vi "Read Array of Message Info.vi"(8 "error in":errorcluster, 11 "Tx execution unit in":refnum<class "Tx Execution Unit.lvclass">) -> (0 "error out":errorcluster, 2 "array of message info":T1[](array[typedef]), 3 "Tx execution unit out":refnum<class "Tx Execution Unit.lvclass">)   [LabVIEW 2020, in "Ballard MIL-STD-1553 Engine.lvlib" / "Implementation.lvlib" / "Tx Execution Unit.lvclass"]
uses:
  Tx Execution Unit.lvclass
  Shared/Tx Write Info.ctl
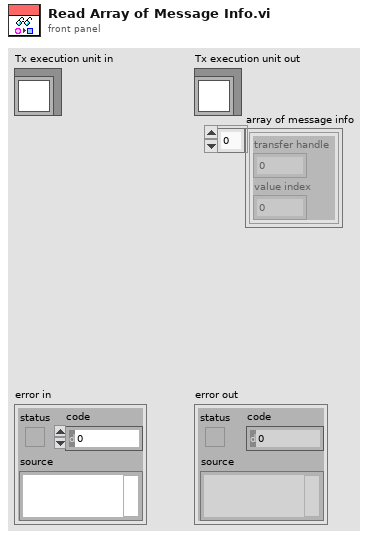
[diagram p1: front panel]
types:
  T1 = typedef "Tx Write Info.ctl" = cluster{"transfer handle":u64, "value index":i32}
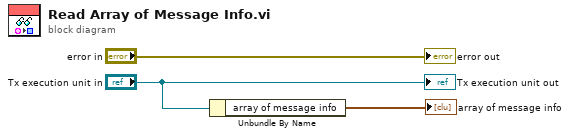
[diagram p0: block diagram]
diagram:
  n1 = Unbundle By Name("Tx execution unit in") -> ("array of message info"=→"array of message info":T1[])
  "error out" <- "error in"
  "Tx execution unit out" <- "Tx execution unit in"
